vi "Get VISA资源名称.vi"(11 "DAM0200-Relay in":refnum<class "DAM0200-Relay.lvclass">) -> (2 "VISA资源名称":refnum<visa-resource-name>, 3 "DAM0200-Relay out":refnum<class "DAM0200-Relay.lvclass">)   [LabVIEW 2016, in "DAM0200-Relay.lvlib" / "DAM0200-Relay.lvclass"]
uses:
  DAM0200-Relay.lvclass
  DAM0200-Relay.lvclass/DAM0200-Relay.ctl
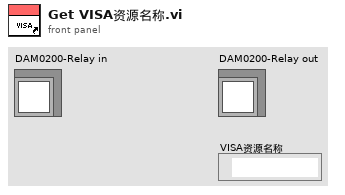
[diagram p1: front panel]
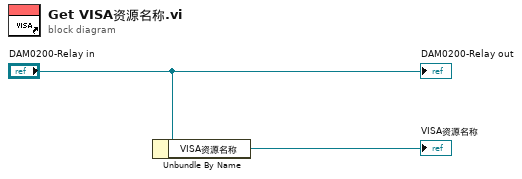
[diagram p0: block diagram]
diagram:
  n1 = Unbundle By Name("DAM0200-Relay in") -> ("VISA资源名称"=→"VISA资源名称":refnum<visa-resource-name>)
  "DAM0200-Relay out" <- "DAM0200-Relay in"
